vi "PWM参数确定.vi"() -> ()   [LabVIEW 2020]
uses:
  62c89ff6-033b-49c9-b5a7-94dd570cd5e2.vi
  ad1d0b6a-49b3-453b-ae3a-4f3b91030ef4.vi
  <vilib>/Array/Sort 2D Array - Pop Stack.vi
  <vilib>/Array/Sort 2D Array - Push Stack.vi
  ad1d0b6a-49b3-453b-ae3a-4f3b91030ef4.vi/269d4b3b-47f5-49e3-8884-44851e4dd9d5.vi
  ad1d0b6a-49b3-453b-ae3a-4f3b91030ef4.vi/6d99389c-673d-4efb-bf33-19b32bcf4cf8.vi
  <vilib>/Comparison/Equal/Equal Functor/Equal Functor.lvclass
panel:
  in  "排序方式":u16(ring) items=["HES", "PLL", "主频", "AHBP", "AHB频率", "占空比分辨率", "实际频率", "相差值", "相差绝对值"]
  in  "+":dbl min=0.0 step=0.1 format="%#_6p"
  out "可选":string[][](table)
  in  "晶振频率":u32=8000000 format="%.0p"
  in  "-":dbl min=0.0 step=0.1 format="%#_6p"
  in  "目标频率":dbl=10000.0 format="%#_6p"
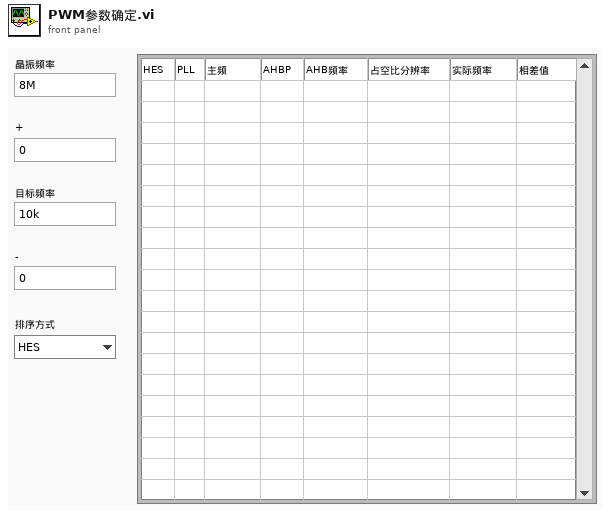
[diagram p1: front panel]
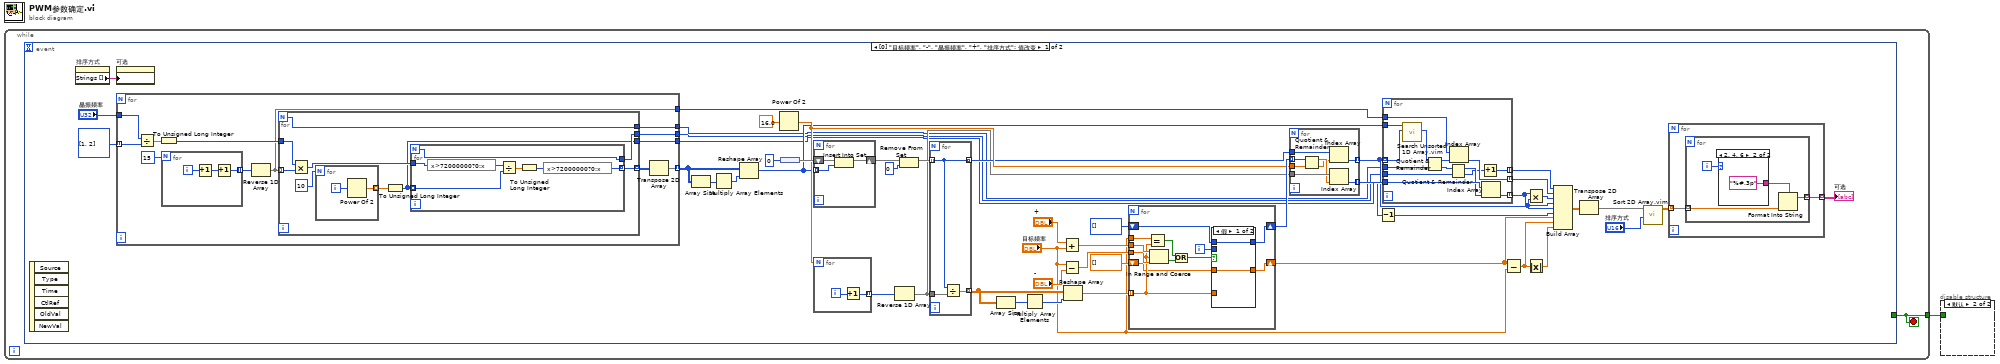
[diagram p0: block diagram]
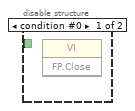
[diagram p2: hidden frame]
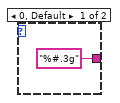
[diagram p3: hidden frame]
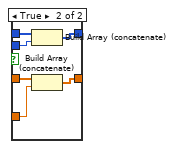
[diagram p4: hidden frame]
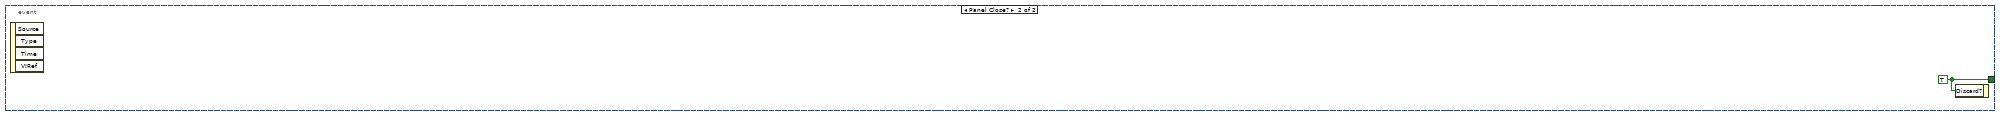
[diagram p5: hidden frame]
diagram:
  n1 = while {
    tunnel: [w2] -> w1
    stop <- w2 stop-if-true
    n2 = event shown="[0] \"目标频率\", \"-\", \"晶振频率\", \"+\", \"排序方式\": 值改变" {
      selector: _ -> [_ _]
      dyn-events: _ -> [_ _]
      timeout: _ -> [_ _]
      tunnel: [_ w142] -> w2
      event "目标频率", "-", "晶振频率", "+", "排序方式": Value Change {
        n3 = event-data() -> ()  [unwired: 1 in, 6 out]
        n4 = property on="排序方式" class="Ring (严格)"() -> ("Strings []"=w7:string[])  [unwired: 2 in, 2 out]
        n5 = property on="可选" class="Tbl (严格)"("Column Headers[]"=w7) -> ()  [unwired: 2 in, 2 out]
        n6 = for {
          tunnel: "晶振频率" -> [w120]
          tunnel: u32[] [1, 2] -> [w119] mode=indexing
          tunnel: [w113] -> w24 mode=indexing
          tunnel: [w112] -> w3
          tunnel: [w111] -> w25
          tunnel: [w110] -> w4
          tunnel: [w109] -> w26
          n7 = Divide(x=w120, y=w119) -> (x/y=w118:dbl)
          n8 = To Unsigned Long Integer(number=w118) -> (unsigned 32bit integer=w117:u32)
          n9 = for {
            N: 15 -> [_]
            tunnel: [w121] -> w116 mode=indexing
            i -> [w123]
            n10 = Increment(x=w123) -> (x+1=w122:i32)
            n11 = Increment(x=w122) -> (x+1=w121:i32)
          }
          n12 = Reverse 1D Array(array=w116) -> (reversed array=w109:i32[])
          n13 = for {
            N -> [w124]
            tunnel: w117 -> [w132]
            tunnel: w109 -> [w131] mode=indexing
            tunnel: [w127] -> w114 mode=indexing
            tunnel: [w126] -> w112
            tunnel: [w125] -> w111
            tunnel: [w124] -> w110
            n14 = Multiply(x=w132, y=w131) -> (x*y=w128:u32)
            n15 = for {
              N: 10 -> [_]
              tunnel: [w140] -> w130 mode=indexing
              i -> [w141]
              n16 = Power Of 2(x=w141) -> (2^x=w140:dbl)
            }
            n17 = To Unsigned Long Integer(number=w130) -> (unsigned 32bit integer=w125:u32[])
            n18 = for {
              N -> [w135]
              tunnel: w125 -> [w137] mode=indexing
              tunnel: w128 -> [w134]
              tunnel: [w136] -> w127 mode=indexing
              tunnel: [w135] -> w126
              n19 = expression code="x>72000000?0:x"(w134) -> (w133:u32)
              n20 = Divide(x=w133, y=w137) -> (x/y=w139:dbl)
              n21 = To Unsigned Long Integer(number=w139) -> (unsigned 32bit integer=w138:u32)
              n22 = expression code="x>72000000?0:x"(w138) -> (w136:u32)
            }
          }
          n23 = Transpose 2D Array(2D array=w114) -> (transposed array=w113:u32[][])
        }
        n24 = Array Size(array=w24) -> (size(s)=w48:i32[])
        n25 = Multiply Array Elements(1:w48) -> (0:w47:i32)
        n26 = Reshape Array(w24, w47) -> (w27:u32[])
        n27 = Power Of 2(x=16.0) -> (2^x=w30:dbl)
        n28 = node(0 ("乘积")) -> (w45:set{i32})
        n29 = for {
          shift-right: [w107] -> w34
          shift-left: w45 -> [w108]
          tunnel: w27 -> [w106] mode=indexing
          n30 = Insert Into Set(10:w106, 11:w108) -> (3:w107:set{i32})  [unwired: 1 out]
        }
        n31 = for {
          N: w30 -> [_]
          tunnel: [w101] -> w43 mode=indexing
          i -> [w102]
          n32 = Increment(x=w102) -> (x+1=w101:i32)
        }
        n33 = Reverse 1D Array(array=w43) -> (reversed array=w28:i32[])
        n34 = Remove From Set(10:0 ("元素"), 11:w34) -> (3:w35:set{i32})  [unwired: 1 out]
        n35 = for {
          tunnel: w35 -> [w103] mode=indexing
          tunnel: [w105] -> w40 mode=indexing
          tunnel: w28 -> [w104]
          tunnel: [w103] -> w29 mode=indexing
          n36 = Divide(x=w103, y=w104) -> (x/y=w105:dbl[])
        }
        n37 = Array Size(array=w40) -> (size(s)=w41:i32[])
        n38 = Multiply Array Elements(1:w41) -> (0:w42:i32)
        n39 = Add(x="+", y="目标频率") -> (x+y=w37:dbl)
        n40 = Subtract(x="目标频率", y="-") -> (x-y=w36:dbl)
        n41 = Reshape Array(w40, w42) -> (w39:dbl[])
        n42 = for {
          tunnel: w39 -> [w83] mode=indexing
          tunnel: w37 -> [w92]
          tunnel: w36 -> [w91]
          shift-right: [w88] -> w31
          shift-left: i32[] [] -> [w87]
          tunnel: "目标频率" -> [w85]
          shift-right: [w82] -> w19
          shift-left: dbl[] [] -> [w81]
          i -> [w89]
          n43 = Equal?(x=w85, y=w83) -> (x = y?=w84:bool)
          n44 = In Range and Coerce(upper limit=w92, x=w83, lower limit=w91) -> (In Range?=w90:bool)  [unwired: 1 out]
          n45 = Or(x=w84, y=w90) -> (x .or. y?=w86:bool)
          n46 = case shown="假" w86 {
            tunnel: w89 -> [_ w100]
            tunnel: [w94 w99] -> w88
            tunnel: w87 -> [w94 w98]
            tunnel: w83 -> [_ w97]
            tunnel: [w93 w96] -> w82
            tunnel: w81 -> [w93 w95]
            frame False {
            }
            frame True {
              n47 = Build Array (concatenate)(w98, w100) -> (w99:i32[])
              n48 = Build Array (concatenate)(w95, w97) -> (w96:dbl[])
            }
          }
        }
        n49 = for {
          tunnel: w31 -> [w80] mode=indexing
          tunnel: w30 -> [w79]
          tunnel: w29 -> [w75]
          tunnel: w28 -> [w78]
          tunnel: [w77] -> w6 mode=indexing
          tunnel: [w73] -> w10 mode=indexing
          n50 = Quotient & Remainder(x=w80, y=w79) -> (x-y*floor(x/y)=w76:dbl, floor(x/y)=w74:dbl)
          n51 = Index Array(array=w75, index=w74) -> (element=w73:i32)
          n52 = Index Array(array=w78, index=w76) -> (element=w77:i32)
        }
        n53 = Decrement(x=w6) -> (x-1=w5:i32[])
        n54 = for {
          tunnel: w10 -> [w72] mode=indexing
          tunnel: w27 -> [w71]
          tunnel: w26 -> [w69]
          tunnel: w25 -> [w66]
          tunnel: [w65] -> w11 mode=indexing
          tunnel: [w68] -> w22 mode=indexing
          tunnel: [w64] -> w23 mode=indexing
          tunnel: w4 -> [w60]
          tunnel: w3 -> [w59]
          n55 = call "Search Unsorted 1D Array.vim"("element"=w72, "unsorted 1D array"=w71) -> ("index of element"=w70:i32)  [unwired: 9 in]
          n56 = Quotient & Remainder(x=w70, y=w60) -> (x-y*floor(x/y)=w63:i32, floor(x/y)=w67:i32)
          n57 = Index Array(array=w69, index=w63) -> (element=w68:i32)
          n58 = Quotient & Remainder(x=w67, y=w59) -> (x-y*floor(x/y)=w62:i32, floor(x/y)=w61:i32)
          n59 = Increment(x=w61) -> (x+1=w64:i32)
          n60 = Index Array(array=w66, index=w62) -> (element=w65:u32)
        }
        n61 = Subtract(x=w19, y="目标频率") -> (x-y=w14:dbl[])
        n62 = Multiply(x=w11, y=w10) -> (x*y=w9:u32[])
        n63 = Absolute Value(x=w14) -> (abs(x)=w13:dbl[])
        n64 = Build Array(w23, w22, w9, w11, w10, w5, w19, w14, w13) -> (w21:dbl[][])
        n65 = Transpose 2D Array(2D array=w21) -> (transposed array=w16:dbl[][])
        n66 = call "Sort 2D Array.vim"("index"="排序方式", "2D array"=w16) -> ("sorted 2D array"=w15:dbl[][])  [unwired: 8 in, 1 out]
        n67 = for {
          tunnel: w15 -> [w52] mode=indexing
          tunnel: [w51] -> w17 mode=indexing
          n68 = for {
            tunnel: w52 -> [w56] mode=indexing
            tunnel: [w54] -> w51 mode=indexing
            i -> [w53]
            n69 = case shown="2, 4, 6" w53 {
              tunnel: ["%#.3g" ("格式字符串") "%#.3p" ("格式字符串")] -> w55
              frame 0, Default {
              }
              frame 2, 4, 6 {
              }
            }
            n70 = Format Into String(format string=w55, w56) -> (resulting string=w54:string)  [unwired: 2 in, 1 out]
          }
        }
        "可选" <- w17
      }
      event Panel Close? {
        w142 = TRUE ("放弃？")
        n71 = event-data() -> ()  [unwired: 1 in, 4 out]
        n72 = event-data("Discard?"=w142) -> ()  [unwired: 1 in, 1 out]
      }
    }
  }
  n73 = disable-structure shown="默认" {
    disable-tunnel: w1 -> [_ _]
    frame condition #0 {
      n74 = invoke class="VI" method="FP.Close"() -> ()  [unwired: 3 in, 3 out]
    }
    frame condition #1 (active) {
    }
  }
